vi "CarWashControls.vi"() -> ()   [LabVIEW 2016, in "test_ValueSignal.lvlib"]
uses:
  test_ValueSignal.lvlib
  example/Car Wash 16.0/Car Wash.vi
  main/apis/Stimulus/ValueSignalByPathString.vi
  main/apis/Assert/AssertControlValueByPathString.vi
  <vilib>/addons/_JKI Toolkits/Caraya/classes/Assert/Assert Equal Value and Type_Variant.vi
  <vilib>/addons/_JKI Toolkits/Caraya/classes/Test/Test.lvclass
  example/Car Wash 16.0/Car Wash.lvlib
  <vilib>/addons/_JKI Toolkits/Caraya/classes/Assert/Assert.lvclass
panel:
  out "error out":errorcluster
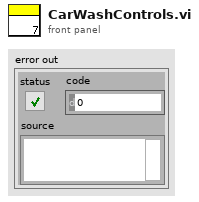
[diagram p1: front panel]
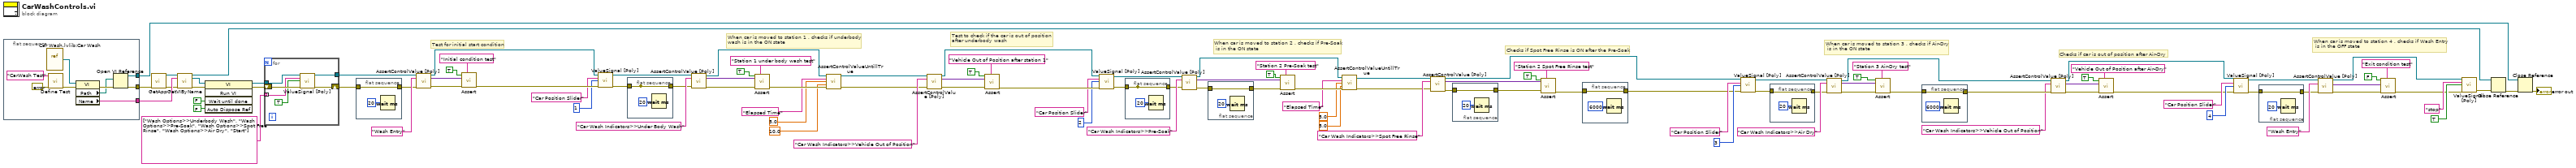
[diagram p0: block diagram]
diagram:
  # "When car is moved to station 4 , checks if Wash Entry\n is in the OFF state"
  # "Checks if car is out of position after Air-Dry"
  # "When car is moved to station 3 , checks if Air-Dry\n is in the ON state"
  # "Checks if Spot Free Rinse is ON after the Pre-Soak"
  # "When car is moved to station 2 , checks if Pre-Soak\n is in the ON state"
  # "Test to check if the car is out of position \nafter underbody wash"
  # "When car is moved to station 1 , checks if underbody \nwash is in the ON state"
  # "Test for initial start condition"
  n1 = flat-sequence {
    tunnel: [w116] -> w110
    tunnel: [w115] -> w16
    tunnel: [w113] -> w109
    frame #0 {
      n2 = vi-ref "Car Wash.lvlib:Car Wash.vi"() -> (w118:refnum<vi>)
      n3 = call <vilib>:"Define Test.vi"("error in (no error)"=errorcluster {"status"=FALSE, "code"=0, "source"=""}, "Label (VI Title)"="CarWash Test") -> ("error out"=w119:errorcluster)  [unwired: 9 in]
      n4 = property on="Property Node" class="VI"(reference=w118, error in=w119) -> (error out=w117:errorcluster, "Path"=w114:path, "Name"=w113:string)  [unwired: 1 out]
      n5 = Open VI Reference(vi path=w114, error in (no error)=w117) -> (vi reference=w115:refnum<vi>, error out=w116:errorcluster)  [unwired: 4 in]
    }
  }
  n6 = call "GetApp.vi"("error in (no error)"=w110) -> ("Application Ref"=w111:refnum<vi>, "error out"=w108:errorcluster)  [unwired: 13 in]
  n7 = call "GetVIByName.vi"("Application Ref in"=w111, "VI Name"=w109, "error in (no error)"=w108) -> ("Application Ref out"=w17:refnum<vi>, "VI Reference"=w105:refnum<vi>, "error out"=w107:errorcluster)  [unwired: 10 in]
  n8 = invoke on="Invoke Node" class="VI" method="Run VI"(reference=w105, error in=w107, "Wait until done"=FALSE ("Wait Until Done"), "Auto Dispose Ref"=FALSE ("Auto Dispose Reference")) -> (reference out=w104:refnum<vi>, error out=w106:errorcluster)  [unwired: 1 in, 3 out]
  n9 = for {
    tunnel: w104 -> [w125]
    tunnel: string[] ["Wash Options>>Underbody Wash", "Wash Options>>Pre-Soak", "Wash Options>>Spot Free Rinse", "Wash Options>>Air Dry", "Start"] -> [w124] mode=indexing
    shift-right: [w122] -> w95
    shift-left: w106 -> [w126]
    tunnel: [w121] -> w93
    n10 = call-poly "ValueSignal [Poly].vi"("VI Reference In"=w125, "Control Name"=w124, "Value (Signaling)"=TRUE, "error in"=w126) -> ("VI Reference Out"=w121:refnum<vi>, "error out"=w122:errorcluster)  [unwired: 10 in]
  }
  n11 = flat-sequence {
    tunnel: w95 -> [w127]
    tunnel: [w127] -> w94
    frame #0 {
      n12 = Wait (ms)(milliseconds to wait=u32 20) -> ()  [unwired: 1 out]
    }
  }
  n13 = call-poly "AssertControlValue [Poly].vi"("VI Reference In"=w93, "Control Name"="Wash Entry", "error in"=w94) -> ("VI Reference Out"=w89:refnum<vi>, "Value"=w98:variant, "error out"=w99:errorcluster)  [unwired: 10 in]
  n14 = call-poly <vilib>:"Assert.vi"("Label"="Initial condition test", "error in (no error)"=w99, "Y"=w98, "X"=TRUE) -> ("error out"=w92:errorcluster)  [unwired: 7 in]
  n15 = call-poly "ValueSignal [Poly].vi"("VI Reference In"=w89, "Control Name"="Car Position Slider", "Value (Signaling)"=u8 1, "error in"=w92) -> ("VI Reference Out"=w88:refnum<vi>, "error out"=w76:errorcluster)  [unwired: 10 in]
  n16 = flat-sequence {
    tunnel: w76 -> [w129]
    tunnel: [w129] -> _
    tunnel: [w129] -> w75
    frame #0 {
      n17 = Wait (ms)(milliseconds to wait=u32 20) -> ()  [unwired: 1 out]
    }
  }
  n18 = call-poly "AssertControlValue [Poly].vi"("VI Reference In"=w88, "Control Name"="Car Wash Indicators>>Under Body Wash", "error in"=w75) -> ("VI Reference Out"=w13:refnum<vi>, "Value"=w83:variant, "error out"=w84:errorcluster)  [unwired: 10 in]
  n19 = call-poly <vilib>:"Assert.vi"("Label"="Station 1 under body wash test", "error in (no error)"=w84, "Y"=w83, "X"=TRUE) -> ("error out"=w14:errorcluster)  [unwired: 7 in]
  n20 = call "AssertControlValueUntillTrue.vi"("VI Reference In"=w13, "Control Name"="Elapsed Time", "Control Value"=5.0, "Timeout(5 sec)"=10.0, "error out"=w14) -> ("VI Reference Out"=w12:refnum<vi>, "error out 2"=w8:errorcluster)  [unwired: 9 in]
  n21 = call-poly "AssertControlValue [Poly].vi"("VI Reference In"=w12, "Control Name"="Car Wash Indicators>>Vehicle Out of Position" ("Label"), "error in"=w8) -> ("VI Reference Out"=w63:refnum<vi>, "Value"=w77:variant, "error out"=w79:errorcluster)  [unwired: 10 in]
  n22 = call-poly <vilib>:"Assert.vi"("Label"="Vehicle Out of Position after station 1", "error in (no error)"=w79, "Y"=w77, "X"=TRUE) -> ("error out"=w78:errorcluster)  [unwired: 7 in]
  n23 = call-poly "ValueSignal [Poly].vi"("VI Reference In"=w63, "Control Name"="Car Position Slider", "Value (Signaling)"=u8 2, "error in"=w78) -> ("VI Reference Out"=w70:refnum<vi>, "error out"=w65:errorcluster)  [unwired: 10 in]
  n24 = flat-sequence {
    tunnel: w65 -> [w131]
    tunnel: [w131] -> _
    tunnel: [w131] -> w64
    frame #0 {
      n25 = Wait (ms)(milliseconds to wait=u32 20) -> ()  [unwired: 1 out]
    }
  }
  n26 = call-poly "AssertControlValue [Poly].vi"("VI Reference In"=w70, "Control Name"="Car Wash Indicators>>Pre-Soak", "error in"=w64) -> ("VI Reference Out"=w5:refnum<vi>, "Value"=w74:variant, "error out"=w67:errorcluster)  [unwired: 10 in]
  n27 = flat-sequence {
    tunnel: w67 -> [w133]
    tunnel: [w133] -> w66
    frame #0 {
      n28 = Wait (ms)(milliseconds to wait=u32 20) -> ()  [unwired: 1 out]
    }
  }
  n29 = call-poly <vilib>:"Assert.vi"("Label"="Station 2 Pre-Soak test", "error in (no error)"=w66, "Y"=w74, "X"=TRUE) -> ("error out"=w7:errorcluster)  [unwired: 7 in]
  n30 = call "AssertControlValueUntillTrue.vi"("VI Reference In"=w5, "Control Name"="Elapsed Time", "Control Value"=5.0, "Timeout(5 sec)"=5.0, "error out"=w7) -> ("VI Reference Out"=w4:refnum<vi>, "error out 2"=w6:errorcluster)  [unwired: 9 in]
  n31 = call-poly "AssertControlValue [Poly].vi"("VI Reference In"=w4, "Control Name"="Car Wash Indicators>>Spot Free Rinse", "error in"=w6) -> ("VI Reference Out"=w45:refnum<vi>, "Value"=w55:variant, "error out"=w59:errorcluster)  [unwired: 10 in]
  n32 = flat-sequence {
    tunnel: w59 -> [w135]
    tunnel: [w135] -> w60
    frame #0 {
      n33 = Wait (ms)(milliseconds to wait=u32 20) -> ()  [unwired: 1 out]
    }
  }
  n34 = call-poly <vilib>:"Assert.vi"("Label"="Station 2 Spot Free Rinse test", "error in (no error)"=w60, "Y"=w55, "X"=TRUE) -> ("error out"=w46:errorcluster)  [unwired: 7 in]
  n35 = flat-sequence {
    tunnel: w46 -> [w137]
    tunnel: [w137] -> w47
    frame #0 {
      n36 = Wait (ms)(milliseconds to wait=u32 6000) -> ()  [unwired: 1 out]
    }
  }
  n37 = call-poly "ValueSignal [Poly].vi"("VI Reference In"=w45, "Control Name"="Car Position Slider", "Value (Signaling)"=u8 3, "error in"=w47) -> ("VI Reference Out"=w50:refnum<vi>, "error out"=w43:errorcluster)  [unwired: 10 in]
  n38 = flat-sequence {
    tunnel: w43 -> [w139]
    tunnel: [w139] -> w42
    frame #0 {
      n39 = Wait (ms)(milliseconds to wait=u32 20) -> ()  [unwired: 1 out]
    }
  }
  n40 = call-poly "AssertControlValue [Poly].vi"("VI Reference In"=w50, "Control Name"="Car Wash Indicators>>Air Dry", "error in"=w42) -> ("VI Reference Out"=w38:refnum<vi>, "Value"=w54:variant, "error out"=w44:errorcluster)  [unwired: 10 in]
  n41 = call-poly <vilib>:"Assert.vi"("Label"="Station 3 Air-Dry test", "error in (no error)"=w44, "Y"=w54, "X"=TRUE) -> ("error out"=w41:errorcluster)  [unwired: 7 in]
  n42 = flat-sequence {
    tunnel: w41 -> [w141]
    tunnel: [w141] -> w40
    frame #0 {
      n43 = Wait (ms)(milliseconds to wait=u32 6000) -> ()  [unwired: 1 out]
    }
  }
  n44 = call-poly "AssertControlValue [Poly].vi"("VI Reference In"=w38, "Control Name"="Car Wash Indicators>>Vehicle Out of Position", "error in"=w40) -> ("VI Reference Out"=w30:refnum<vi>, "Value"=w35:variant, "error out"=w36:errorcluster)  [unwired: 10 in]
  n45 = call-poly <vilib>:"Assert.vi"("Label"="Vehicle Out of Position after Air-Dry", "error in (no error)"=w36, "Y"=w35, "X"=TRUE) -> ("error out"=w31:errorcluster)  [unwired: 7 in]
  n46 = call-poly "ValueSignal [Poly].vi"("VI Reference In"=w30, "Control Name"="Car Position Slider", "Value (Signaling)"=u8 4, "error in"=w31) -> ("VI Reference Out"=w29:refnum<vi>, "error out"=w21:errorcluster)  [unwired: 10 in]
  n47 = flat-sequence {
    tunnel: w21 -> [w143]
    tunnel: [w143] -> _
    tunnel: [w143] -> w20
    frame #0 {
      n48 = Wait (ms)(milliseconds to wait=u32 20) -> ()  [unwired: 1 out]
    }
  }
  n49 = call-poly "AssertControlValue [Poly].vi"("VI Reference In"=w29, "Control Name"="Wash Entry", "error in"=w20) -> ("VI Reference Out"=w22:refnum<vi>, "Value"=w24:variant, "error out"=w25:errorcluster)  [unwired: 10 in]
  n50 = call-poly <vilib>:"Assert.vi"("Label"="Exit condition test", "error in (no error)"=w25, "Y"=w24, "X"=FALSE) -> ("error out"=w23:errorcluster)  [unwired: 7 in]
  n51 = call-poly "ValueSignal [Poly].vi"("VI Reference In"=w22, "Control Name"="stop", "Value (Signaling)"=TRUE, "error in"=w23) -> ("error out"=w19:errorcluster)  [unwired: 10 in, 1 out]
  n52 = Close Reference(reference=w17, error in (no error)=w19) -> (error out=w18:errorcluster)
  n53 = Close Reference(reference=w16, error in (no error)=w18) -> (error out=→"error out":errorcluster)
